vi "Init PWM Waveform DVRs.vi"(8 "error in":errorcluster, 11 "DO DAQmx Fixed Freq PWM CFG in":refnum<class "DO DAQmx Fixed Freq PWM CFG.lvclass">) -> (0 "error out":errorcluster, 3 "DO DAQmx Fixed Freq PWM CFG out":refnum<class "DO DAQmx Fixed Freq PWM CFG.lvclass">)   [LabVIEW 2023, in "DO DAQmx Fixed Freq PWM CFG.lvclass"]
uses:
  DO DAQmx Fixed Freq PWM CFG.lvclass
  DO DAQmx Fixed Freq PWM CFG.lvclass/DO DAQmx Fixed Freq PWM CFG.ctl
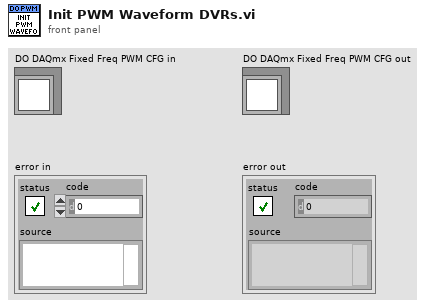
[diagram p1: front panel]
types:
  T1 = cluster{"Channel":string, "Digital Waveform":digitalwaveform}[]
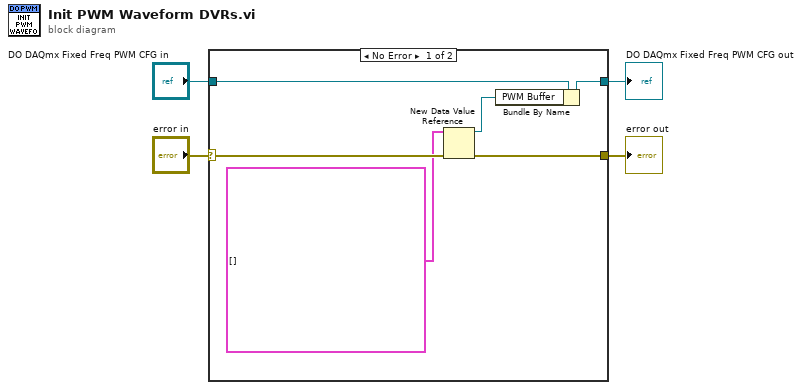
[diagram p0: block diagram]
diagram:
  n1 = case shown="No Error" "error in" {
    selector: "error in" -> [w8 w12]
    tunnel: [w7 w12] -> w3
    tunnel: [w9 w11] -> w1
    tunnel: "DO DAQmx Fixed Freq PWM CFG in" -> [w10 w11]
    frame No Error {
      n2 = New Data Value Reference(data value=T1 [] ("PWM Buffer"), error in=w8) -> (data value reference=w5:refnum<data-value>, error out=w7:errorcluster)
      n3 = Bundle By Name(cluster=w10, "PWM Buffer"=w5) -> (w9:refnum<class "DO DAQmx Fixed Freq PWM CFG.lvclass">)
    }
    frame Error {
    }
  }
  "error out" <- w3
  "DO DAQmx Fixed Freq PWM CFG out" <- w1
